vi "Drive Immediate.vi"(4 "80A(T)/45(F)":bool, 5 "Operation":T1, 6 "Synchronication":enum16{"Start", "Wait"}(ring), 7 "Description":string, 8 "Command Info In":T3, 9 "Modifiers":T2={"Reverse (T) / Normal (F)"=FALSE, "Power Scaling (1=Normal) "=1.0, "Deadband Value"=0.01}, 10 "Right Setpoint (Turning)":dbl, 11 "Left Setpoint (Power)":dbl) -> (0 "Command Info Out":T3)   [LabVIEW 2018]
doc: "Often used for joystick control, this VI checks to see that the joystick axes are outside the deadband and updates the motors appropriately."
uses:
  <vilib>/Rock Robotics/WPI/Framework/Command Status Info.ctl
  <vilib>/Rock Robotics/WPI/Framework/Completion Status.ctl
  <vilib>/Rock Robotics/WPI/Framework/Completion Notifier.ctl
  Implementation/Drive Operations.ctl
  Implementation/Drive Setpoints.ctl
  Support Code/Path Data.ctl
  Support Code/Availible Command systems for auto.ctl
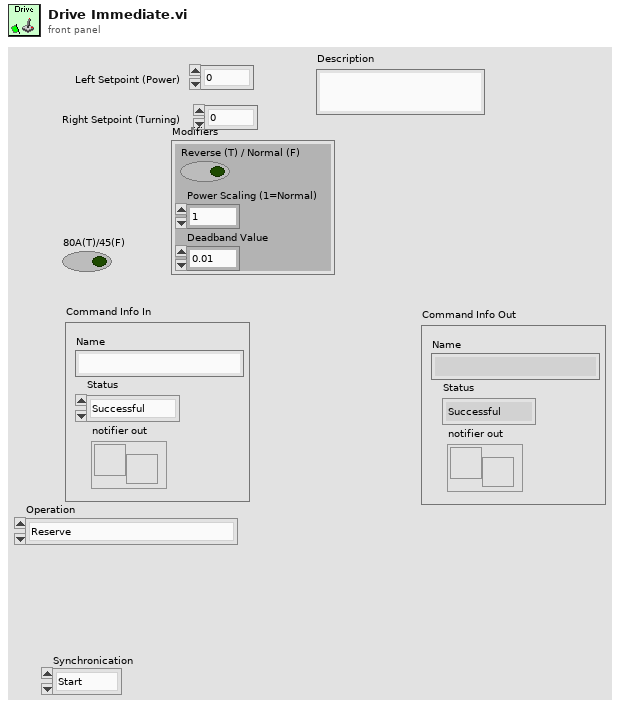
[diagram p1: front panel]
types:
  T1 = typedef "Drive Operations.ctl" = enum16{"Reserve", "Read Current", "Immediate", "J-Turn", "Play Back From Log", "Auto-Align"}
  T2 = cluster{"Reverse (T) / Normal (F)":bool, "Power Scaling (1=Normal) ":dbl, "Deadband Value":dbl}
  T3 = typedef "Command Status Info.ctl" = cluster{"Name":string, "Status":T4, "notifier out":T5}
  T4 = typedef "Completion Status.ctl" = enum16{"Successful", "Aborted", "Incomplete"}
  T5 = typedef "Completion Notifier.ctl" = refnum<notifier>
  T6 = typedef "Drive Setpoints.ctl" = cluster{"Operation":T1, "Left Setpoint (Power)":dbl, "Right Setpoint (Turning)":dbl, "Reverse (T) / Normal (F)":bool, "Power Scaling (1=Normal) ":dbl, "Path Data":T7, "Path":path, "Angle boi":dbl, "Path Reversed":bool, "Align for Path":bool, "80A(T)/45(F)":bool, "Auto Path Data":cluster{"V":dbl[], "Theta":dbl[], "Commands":cluster{"Time into Path":dbl, "System":T8, "Item Selected?":bool, "System Selection":T8}[], "Sample Period":dbl}}
  T7 = typedef "Path Data.ctl" = cluster{"Maneuver":enum16{"MAX 90", "MAX 180", "Turn to Home", "Turn to Rocket", "Auto-Align", "Turn to ..."}, "Rotation Direction":enum16{"N/A", "Right", "Left"}}[]
  T8 = typedef "Availible Command systems for auto.ctl" = u16
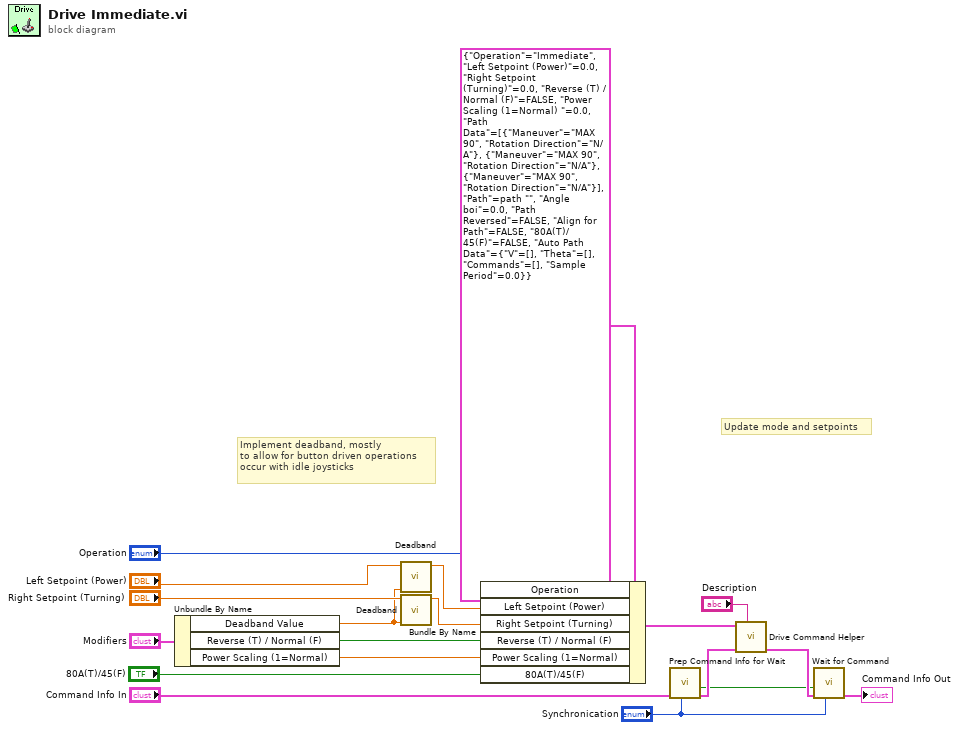
[diagram p0: block diagram]
diagram:
  # "Implement deadband, mostly\nto allow for button driven operations\noccur with idle joysticks"
  # "Update mode and setpoints"
  n1 = Unbundle By Name("Modifiers") -> ("Deadband Value"=w12:dbl, "Reverse (T) / Normal (F)"=w11:bool, "Power Scaling (1=Normal)"=w10:dbl)
  n2 = call "Deadband.vi"("Deadband"=w12, "Input"="Left Setpoint (Power)") -> ("f"=w15:dbl)  [unwired: 9 in]
  n3 = call "Deadband.vi"("Deadband"=w12, "Input"="Right Setpoint (Turning)") -> ("f"=w14:dbl)  [unwired: 9 in]
  n4 = Bundle By Name(cluster=T6 {"Operation"=enum."Immediate", "Left Setpoint (Power)"=0.0, "Right Setpoint (Turning)"=0.0, "Reverse (T) / Normal (F)"=FALSE, "Power Scaling (1=Normal) "=0.0, "Path Data"=[{"Maneuver"=enum."MAX 90", "Rotation Direction"=enum."N/A"}, {"Maneuver"=enum."MAX 90", "Rotation Direction"=enum."N/A"}, {"Maneuver"=enum."MAX 90", "Rotation Direction"=enum."N/A"}], "Path"=path "", "Angle boi"=0.0, "Path Reversed"=FALSE, "Align for Path"=FALSE, "80A(T)/45(F)"=FALSE, "Auto Path Data"={"V"=[], "Theta"=[], "Commands"=[], "Sample Period"=0.0}} ("SubSystem Data"), "Operation"="Operation", "Left Setpoint (Power)"=w15, "Right Setpoint (Turning)"=w14, "Reverse (T) / Normal (F)"=w11, "Power Scaling (1=Normal)"=w10, "80A(T)/45(F)"="80A(T)/45(F)") -> (w17:T6)
  n5 = call <vilib>:"Prep Command Info for Wait.vi"("Synchronication"="Synchronication", "Command Info"="Command Info In") -> ("Command Info"=w7:T3, "Allocated"=w4:bool)  [unwired: 8 in]
  n6 = call "Drive Command Helper.vi"("Description"="Description", "Command Info In"=w7, "SubSystem Data"=w17) -> ("Command Info Out"=w6:T3)  [unwired: 6 in, 2 out]
  n7 = call <vilib>:"Wait for Command.vi"("Synchronication"="Synchronication", "Command Info in"=w6, "Allocated"=w4) -> ("Command Info out"=→"Command Info Out":T3)  [unwired: 8 in]
